vi "get_temporary_file_folder.vi"(8 "error in (no error)":errorcluster, 11 "ImageCollection.lvclass in":refnum<class "ImageCollection.lvclass">) -> (0 "error out":errorcluster, 2 "temporary file folder":path, 3 "ImageCollection.lvclass out":refnum<class "ImageCollection.lvclass">)   [LabVIEW 2010, in "ImageCollection.lvclass"]
uses:
  ImageCollection.lvclass
  ImageCollection.lvclass/ImageCollection.ctl
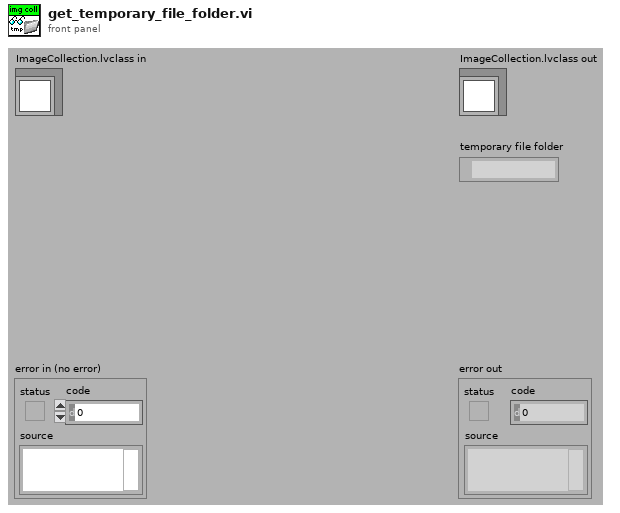
[diagram p1: front panel]
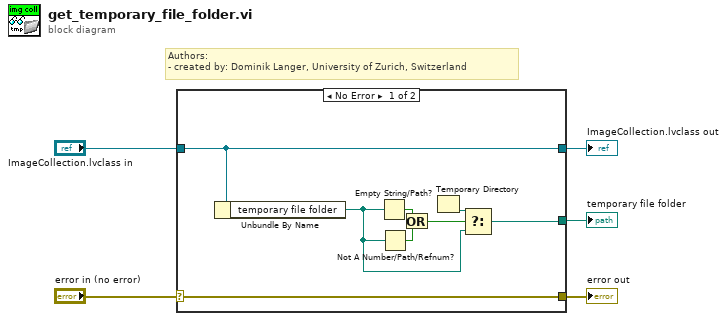
[diagram p0: block diagram]
diagram:
  # "Authors: \n- created by: Dominik Langer, University of Zurich, Switzerland"
  n1 = case shown="No Error" "error in (no error)" {
    selector: "error in (no error)" -> [w13 w14]
    tunnel: [w13 w14] -> w4
    tunnel: [w12 w15] -> w2
    tunnel: "ImageCollection.lvclass in" -> [w12 w15]
    tunnel: [w6 _] -> w1
    frame No Error {
      n2 = Unbundle By Name(w12) -> ("temporary file folder"=w7:path)
      n3 = Empty String/Path?(string/path=w7) -> (empty?=w9:bool)
      n4 = Not A Number/Path/Refnum?(number/path/refnum=w7) -> (NaN/Path/Refnum?=w10:bool)
      n5 = Or(x=w9, y=w10) -> (x .or. y?=w11:bool)
      n6 = Temporary Directory() -> (w8:path)
      n7 = Select(t=w8, s=w11, f=w7) -> (s? t:f=w6:path)
    }
    frame Error {
    }
  }
  "error out" <- w4
  "ImageCollection.lvclass out" <- w2
  "temporary file folder" <- w1
